vi "Latest.vi"(7 "LabVIEW Web Service Request":refnum<class "Web Request.lvclass">) -> ()   [LabVIEW 2023]
uses:
  <vilib>/wsapi/Web Request.lvclass
panel:
  # "Use the Web Service Request input terminal to call the VIs on the Web Services palette. Do not remove it from the connector pane unless you don't need access to the palette."
  # "Each additional control wired to the connector pane will be available as an input in the URL. To include an indicator in terminal-mode output (the default setting), it must also be wired to the connector pane."
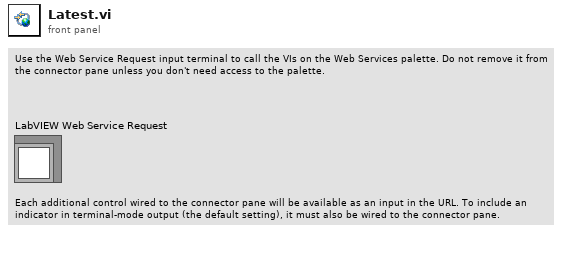
[diagram p1: front panel]
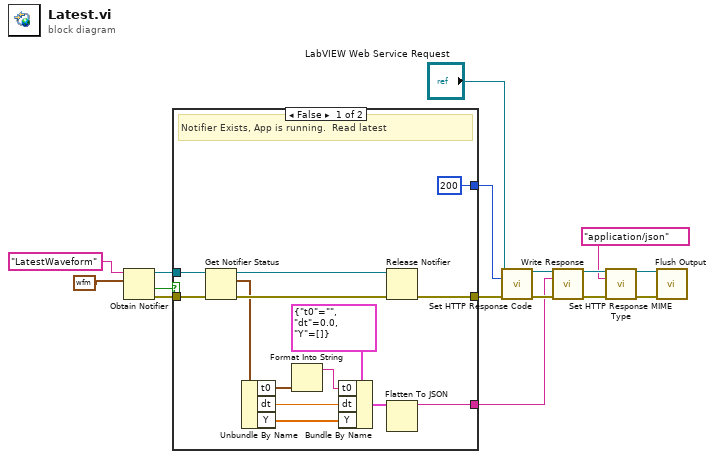
[diagram p0: block diagram]
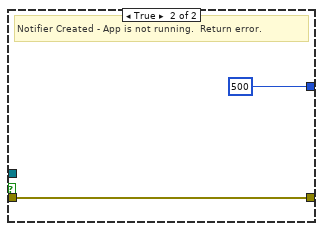
[diagram p2: hidden frame]
diagram:
  n1 = Obtain Notifier(name (unnamed)="LatestWaveform", notification data type=waveform(dbl) {"t0"=timestamp(0 s since 1904-01-01), "dt"=1.0, "Y"=[]}) -> (notifier out=w14:refnum<notifier>, created new?=w6:bool, error out=w13:errorcluster)  [unwired: 2 in]
  n2 = case shown="False" w6 {
    tunnel: w14 -> [w29 _]
    tunnel: w13 -> [w28 w32]
    tunnel: [w25 w32] -> w10
    tunnel: [200 500] -> w8
    tunnel: [w17 _] -> w7
    frame False {
      # "Notifier Exists, App is running.  Read latest"
      n3 = Get Notifier Status(notifier=w29, error in (no error)=w28) -> (notifier out=w26:refnum<notifier>, current notification=w24:waveform(dbl), error out=w27:errorcluster)  [unwired: 2 out]
      n4 = Unbundle By Name(w24) -> ("t0"=w21:timestamp, "dt"=w23:dbl, "Y"=w22:dbl[])
      n5 = Format Into String(w21) -> (resulting string=w20:string)  [unwired: 3 in, 1 out]
      n6 = Bundle By Name(cluster=cluster{"t0":string, "dt":dbl, "Y":dbl[]} {"t0"="", "dt"=0.0, "Y"=[]}, "t0"=w20, "dt"=w23, "Y"=w22) -> (w18:cluster{"t0":string, "dt":dbl, "Y":dbl[]})
      n7 = Release Notifier(notifier=w26, error in (no error)=w27) -> (error out=w25:errorcluster)  [unwired: 1 in, 2 out]
      n8 = Flatten To JSON(anything=w18) -> (JSON string=w17:string)  [unwired: 2 in, 1 out]
    }
    frame True {
      # "Notifier Created - App is not running.  Return error."
    }
  }
  n9 = call <vilib>:"Set HTTP Response Code.vi"("LabVIEW Web Service Request"="LabVIEW Web Service Request", "response code (200)"=w8, "error in (no error)"=w10) -> ("LabVIEW Web Service Request out"=w12:refnum<class "Web Request.lvclass">, "error out"=w11:errorcluster)  [unwired: 11 in]
  n10 = call <vilib>:"Write Response.vi"("LabVIEW Web Service Request"=w12, "response string"=w7, "error in (no error)"=w11) -> ("LabVIEW Web Service Request out"=w5:refnum<class "Web Request.lvclass">, "error out"=w4:errorcluster)  [unwired: 11 in]
  n11 = call <vilib>:"Set HTTP Response MIME Type.vi"("LabVIEW Web Service Request"=w5, "MIME type (text/html)"="application/json", "error in (no error)"=w4) -> ("LabVIEW Web Service Request out"=w2:refnum<class "Web Request.lvclass">, "error out"=w3:errorcluster)  [unwired: 11 in]
  n12 = call <vilib>:"Flush Output.vi"("LabVIEW Web Service Request"=w2, "error in (no error)"=w3) -> ()  [unwired: 12 in, 2 out]
